vi "String to ASCII Code.vi"(10 "String":string) -> (1 "Array - String":string[](array[string]), 2 "Array of ASCII Codes":u8[](array[numeric]) format="%.0f        0x%.0x")   [LabVIEW 2016]
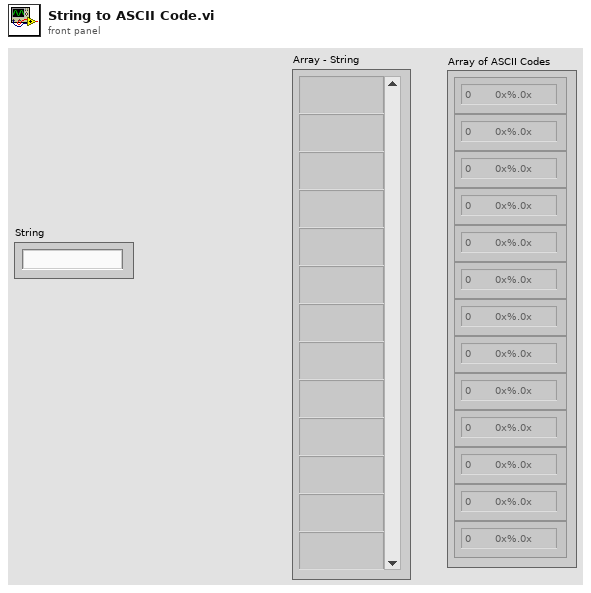
[diagram p1: front panel]
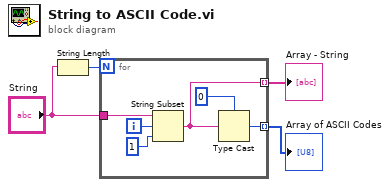
[diagram p0: block diagram]
diagram:
  n1 = String Length(string="String") -> (length=w4:i32)
  n2 = for {
    N: w4 -> [_]
    tunnel: "String" -> [w10]
    tunnel: [w6] -> w2 mode=indexing
    tunnel: [w5] -> w3 mode=indexing
    i -> [w9]
    n3 = String Subset(string=w10, offset (0)=w9, length (rest)=1 ("length (rest)")) -> (substring=w6:string)
    n4 = Type Cast(type=i8 0, x=w6) -> (*(type *) &x=w5:i8)
  }
  "Array of ASCII Codes" <- w3
  "Array - String" <- w2
